vi "Read Thermocouple Type.vi"(8 "error in (no error)":errorcluster, 11 "BNT_DMQmx-MCSV-TC in":refnum<class "BNT_DMQmx-MCSV-TC.lvclass">) -> (0 "error out":errorcluster, 2 "Thermocouple Type":i32(ring)=10072 items=["J"=10072, "K"=10073, "N"=10077, "R"=10082, "S"=10085, "T"=10086, "B"=10047, "E"=10055], 3 "BNT_DMQmx-MCSV-TC out":refnum<class "BNT_DMQmx-MCSV-TC.lvclass">)   [LabVIEW 2016, in "BNT_DAQmx.lvlib" / "BNT_DMQmx-MCSV-TC.lvclass"]
doc: "Read Thermocouple Type."
uses:
  BNT_DMQmx-MCSV-TC.lvclass
  BNT_DMQmx-MCSV-TC.lvclass/BNT_DMQmx-MCSV-TC.ctl
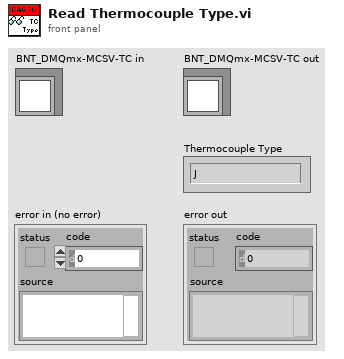
[diagram p1: front panel]
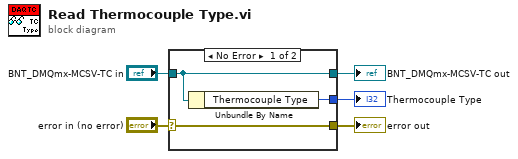
[diagram p0: block diagram]
diagram:
  n1 = case shown="No Error" "error in (no error)" {
    selector: "error in (no error)" -> [w8 w9]
    tunnel: [w8 w9] -> w4
    tunnel: [w7 w10] -> w2
    tunnel: "BNT_DMQmx-MCSV-TC in" -> [w7 w10]
    tunnel: [w6 _] -> w1
    frame No Error {
      n2 = Unbundle By Name(w7) -> ("Thermocouple Type"=w6:i32)
    }
    frame Error {
    }
  }
  "error out" <- w4
  "BNT_DMQmx-MCSV-TC out" <- w2
  "Thermocouple Type" <- w1
